vi "X_4352_Y.vi"(0 "x0":dbl format="%#_13g", 5 "x1":dbl format="%#_13g", 7 "x2":dbl format="%#_13g", 9 "x3":dbl format="%#_13g", 11 "x4":dbl format="%#_13g", 12 "e":dbl format="%#_13g", 13 "q0":dbl format="%#_13g", 14 "qzsum":dbl format="%#_13g") -> (8 "Yout":dbl)   [LabVIEW 2019]
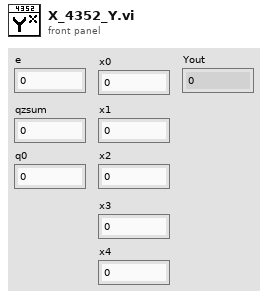
[diagram p1: front panel]
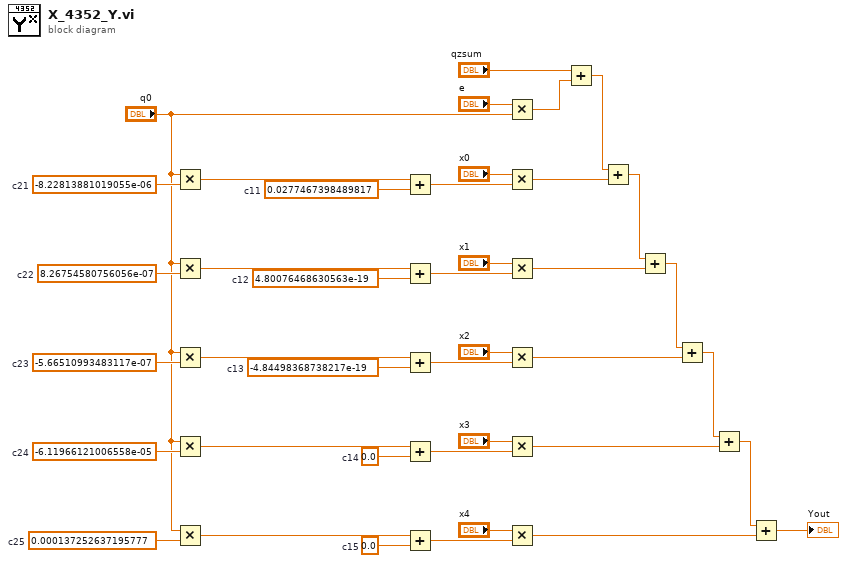
[diagram p0: block diagram]
diagram:
  w34 = 0.0277467398489817  # c11
  w30 = -4.84498368738217e-19  # c13
  w26 = 0.0  # c15
  w28 = 0.0  # c14
  w32 = 4.80076468630563e-19  # c12
  w36 = -8.22813881019055e-06  # c21
  w38 = -5.66510993483117e-07  # c23
  w40 = 0.000137252637195777  # c25
  w39 = -6.11966121006558e-05  # c24
  w37 = 8.26754580756056e-07  # c22
  n1 = Multiply(x="q0", y=w36) -> (x*y=w35:dbl)
  n2 = Multiply(x="q0", y=w37) -> (x*y=w33:dbl)
  n3 = Multiply(x="q0", y=w38) -> (x*y=w31:dbl)
  n4 = Multiply(x="q0", y=w39) -> (x*y=w29:dbl)
  n5 = Multiply(x="q0", y=w40) -> (x*y=w27:dbl)
  n6 = Add(x=w35, y=w34) -> (x+y=w22:dbl)
  n7 = Add(x=w33, y=w32) -> (x+y=w23:dbl)
  n8 = Add(x=w31, y=w30) -> (x+y=w24:dbl)
  n9 = Add(x=w29, y=w28) -> (x+y=w5:dbl)
  n10 = Add(x=w27, y=w26) -> (x+y=w25:dbl)
  n11 = Multiply(x="e", y="q0") -> (x*y=w6:dbl)
  n12 = Multiply(x="x0", y=w22) -> (x*y=w12:dbl)
  n13 = Multiply(x="x1", y=w23) -> (x*y=w11:dbl)
  n14 = Multiply(x="x2", y=w24) -> (x*y=w10:dbl)
  n15 = Multiply(x="x3", y=w5) -> (x*y=w9:dbl)
  n16 = Multiply(x="x4", y=w25) -> (x*y=w7:dbl)
  n17 = Add(x="qzsum", y=w6) -> (x+y=w14:dbl)
  n18 = Add(x=w14, y=w12) -> (x+y=w16:dbl)
  n19 = Add(x=w16, y=w11) -> (x+y=w13:dbl)
  n20 = Add(x=w13, y=w10) -> (x+y=w15:dbl)
  n21 = Add(x=w15, y=w9) -> (x+y=w8:dbl)
  n22 = Add(x=w8, y=w7) -> (x+y=→"Yout":dbl)
